vi "DAQmxSin INIT.vi"(7 "physical channels":tag="Dev2/ao0", 8 "error in":errorcluster, 10 "sine wave":dbl[](array[numeric]), 11 "DAQmxChannel":T1) -> (0 "error out":errorcluster, 3 "task out":refnum<k21>)   [LabVIEW 2020]
uses:
  <vilib>/DAQmx/write.llb/DAQmx Write (Analog Wfm 1Chan NSamp).vi
  <vilib>/DAQmx/create/channels.llb/DAQmx Create Channel (AO-Voltage-Basic).vi
  <vilib>/DAQmx/configure/timing.llb/DAQmx Timing (Sample Clock).vi
  <vilib>/DAQmx/miscellaneous.llb/DAQmx Fill In Error Info.vi
panel:
  out "number of samples written per channel":u32
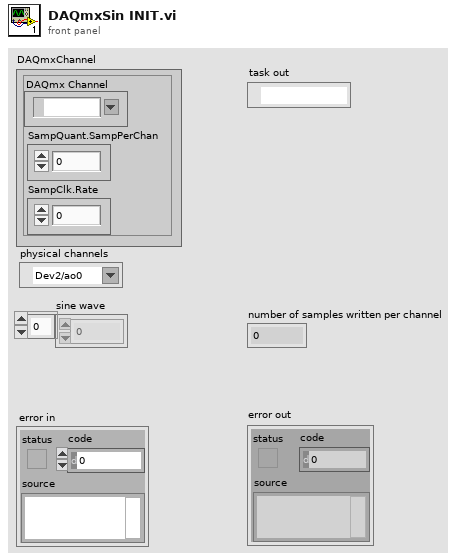
[diagram p1: front panel]
types:
  T1 = cluster{"SampClk.Rate":dbl, "SampQuant.SampPerChan":i32, "DAQmx Channel":refnum<k21>}
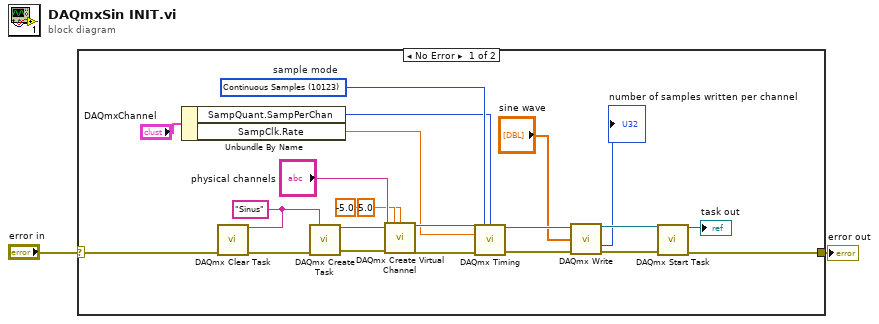
[diagram p0: block diagram]
diagram:
  n1 = case shown="No Error" "error in" {
    selector: "error in" -> [w15 w25]
    tunnel: [w23 w25] -> w2
    frame No Error {
      w13 = "Sinus" ("task name")
      w24 = 10123 items=["Finite Samples"=10178, "Continuous Samples"=10123, "Hardware Timed Single Point"=12522]  # sample mode
      n2 = Unbundle By Name("DAQmxChannel") -> ("SampQuant.SampPerChan"=w12:i32, "SampClk.Rate"=w11:dbl)
      n3 = call <vilib>:"DAQmx Clear Task.vi"("task in"=w13, "error in"=w15) -> ("error out"=w14:errorcluster)  [unwired: 13 in]
      n4 = call <vilib>:"DAQmx Create Task.vi"("new task name"=w13, "error in"=w14) -> ("task out"=w20:refnum<k21>, "error out"=w17:errorcluster)  [unwired: 12 in]
      n5 = call-poly <vilib>:"DAQmx Create Virtual Channel.vi"("task in"=w20, "maximum value"=5.0, "minimum value"=-5.0, "physical channels"="physical channels", "error in"=w17) -> ("task out"=w19:refnum<k21>, "error out"=w18:errorcluster)  [unwired: 9 in]
      n6 = call-poly <vilib>:"DAQmx Timing.vi"("task/channels in"=w19, "sample mode"=w24, "samples per channel"=w12, "rate"=w11, "error in"=w18) -> ("task out"=w10:refnum<k21>, "error out"=w8:errorcluster)  [unwired: 9 in]
      n7 = call-poly <vilib>:"DAQmx Write.vi"("task/channels in"=w10, "data"="sine wave", "error in"=w8) -> ("task out"=w9:refnum<k21>, "number of samples written per channel"=→"number of samples written per channel":u32, "error out"=w7:errorcluster)  [unwired: 10 in]
      n8 = call <vilib>:"DAQmx Start Task.vi"("task/channels in"=w9, "error in"=w7) -> ("task out"=→"task out":refnum<k21>, "error out"=w23:errorcluster)  [unwired: 12 in]
    }
    frame Error {
    }
  }
  "error out" <- w2
